vi "Asia Pump C Test.vi"() -> ()   [LabVIEW 2018, in "ASIA Pump.lvlib"]
uses:
  ASIA Pump.lvlib
  ASIA Pump/Pump Settings.ctl
panel:
  out "ASIA Pump Global 2":T1(array[cluster])
  out "ASIA Pump Global":T1(array[cluster])
  out "Set Speed Connection error":bool
  out "scan error out":errorcluster
  out "Initialized":bool
  out "No Pump Connected":bool=TRUE
  out "Enter Remote Completed":bool=TRUE
  in  "Enum":T2(ring)
  in  "stop 3":bool
  out "Set Overpressure Strategy":bool
  out "pumpCnt":u32
  in  "ASIA Pump C Settings in 3":T3={"ASIA Pump #"=0, "channel"=1, "Simulated"=FALSE}
  out "Pump On?":enum16{"Off", "On", "Not Initialized"}(ring)
  out "pressure":dbl
  out "Connection Error 2":bool
  out "Connection Error":bool
  out "Pump Status Time":dbl
  out "Set Speed Time":dbl
  in  "Pump %":sgl
  in  "stop":bool
  out "PumpStatusCode":T4(ring)=enum."Idle"
  out "pumpRate":dbl format="%.2f"
  out "syringeSize":sgl
  in  "Run":bool
  in  "ASIA Pump C Settings in":T3
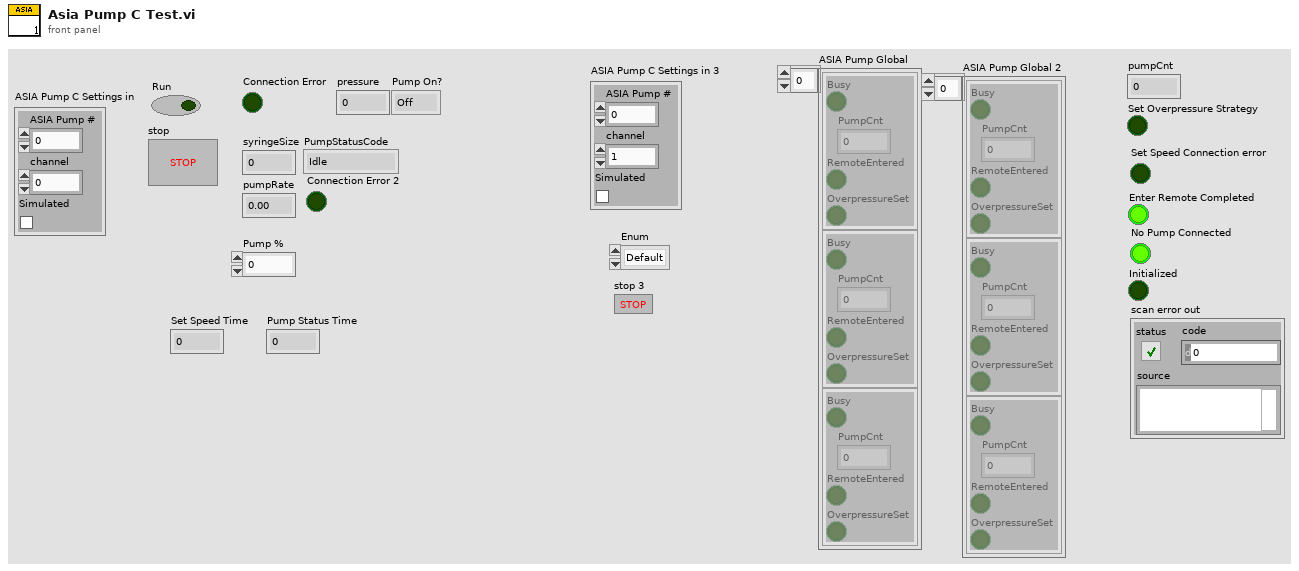
[diagram p1: front panel]
types:
  T1 = cluster{"Busy":bool, "PumpCnt":dbl, "RemoteEntered":bool, "OverpressureSet":bool}[]
  T2 = enum16{"Default", "EnterRemote", "Scan", "overpress", "initialize", "pump"}
  T3 = typedef "ASIA Pump.lvlib/Pump Settings.ctl" = cluster{"ASIA Pump #":i32, "channel":i32, "Simulated":bool}
  T4 = enum16{"Error", "Uninitialised", "Initialising", "Idle", "Filling", "Full", "Emptying", "Empty", "Pumping", "Default"}
  T5 = enum16{"Default", "EnterRemote", "Scan", "overpress"}
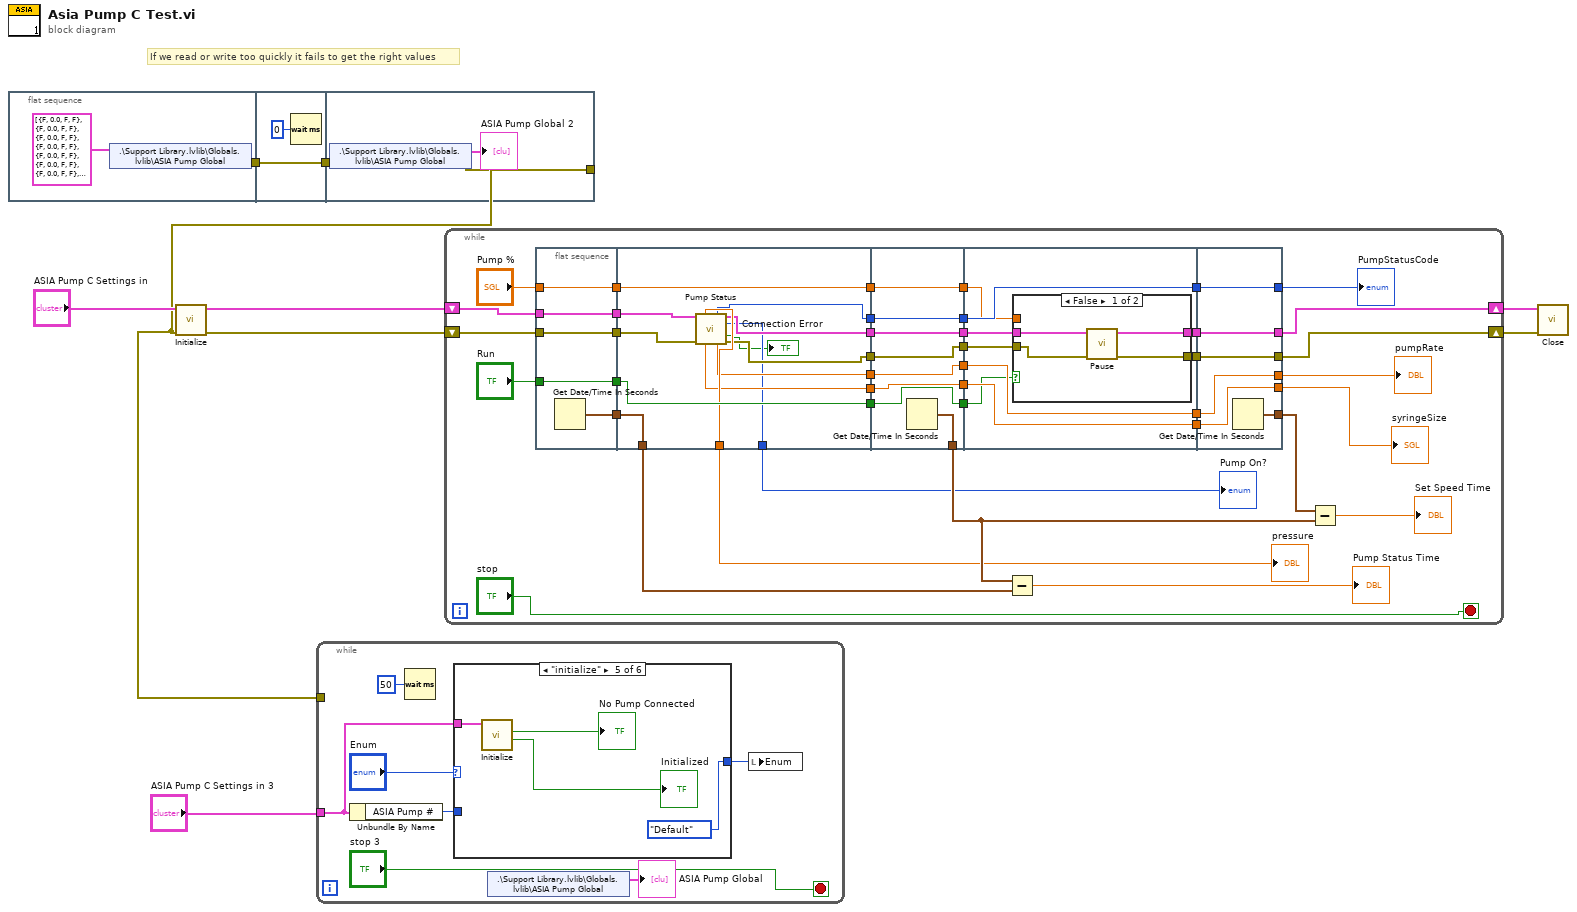
[diagram p0: block diagram]
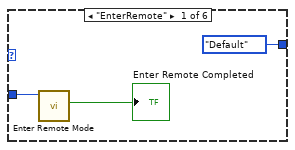
[diagram p2: hidden frame]
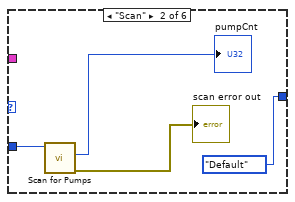
[diagram p3: hidden frame]
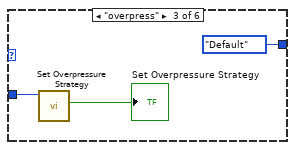
[diagram p4: hidden frame]
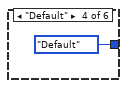
[diagram p5: hidden frame]
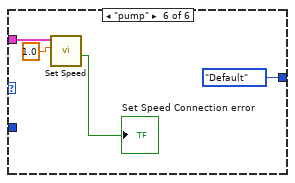
[diagram p6: hidden frame]
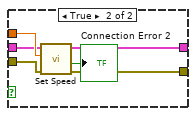
[diagram p7: hidden frame]
diagram:
  # "If we read or write too quickly it fails to get the right values"
  n1 = flat-sequence {
    tunnel: [w10] -> w3
    tunnel: w3 -> [w13]
    tunnel: [w13] -> w2
    tunnel: w2 -> [w15]
    tunnel: [w14] -> w1
    frame #0 {
      n2 = shared-variable ".\\Support Library.lvlib\\Globals.lvlib\\ASIA Pump Global"(T1 [{"Busy"=FALSE, "PumpCnt"=0.0, "RemoteEntered"=FALSE, "OverpressureSet"=FALSE}, {"Busy"=FALSE, "PumpCnt"=0.0, "RemoteEntered"=FALSE, "OverpressureSet"=FALSE}, {"Busy"=FALSE, "PumpCnt"=0.0, "RemoteEntered"=FALSE, "OverpressureSet"=FALSE}, {"Busy"=FALSE, "PumpCnt"=0.0, "RemoteEntered"=FALSE, "OverpressureSet"=FALSE}, {"Busy"=FALSE, "PumpCnt"=0.0, "RemoteEntered"=FALSE, "OverpressureSet"=FALSE}, {"Busy"=FALSE, "PumpCnt"=0.0, "RemoteEntered"=FALSE, "OverpressureSet"=FALSE}, {"Busy"=FALSE, "PumpCnt"=0.0, "RemoteEntered"=FALSE, "OverpressureSet"=FALSE}, {"Busy"=FALSE, "PumpCnt"=0.0, "RemoteEntered"=FALSE, "OverpressureSet"=FALSE}, {"Busy"=FALSE, "PumpCnt"=0.0, "RemoteEntered"=FALSE, "OverpressureSet"=FALSE}, {"Busy"=FALSE, "PumpCnt"=0.0, "RemoteEntered"=FALSE, "OverpressureSet"=FALSE}, {"Busy"=FALSE, "PumpCnt"=0.0, "RemoteEntered"=FALSE, "OverpressureSet"=FALSE}] ("ASIA Pump Global")) -> (error out=w10:errorcluster)  [unwired: 1 in]
    }
    frame #1 {
      n3 = Wait (ms)(milliseconds to wait=u32 0) -> ()  [unwired: 1 out]
    }
    frame #2 {
      n4 = shared-variable ".\\Support Library.lvlib\\Globals.lvlib\\ASIA Pump Global"(error in=w15) -> (→"ASIA Pump Global 2":T1, error out=w14:errorcluster)
    }
  }
  n5 = call "Initialize.vi"("error in (no error)"=w1, "ASIA Pump C Settings in"="ASIA Pump C Settings in") -> ("error out"=w5:errorcluster, "ASIA Pump C Settings out"=w8:T3)  [unwired: 6 in, 2 out]
  n6 = while {
    tunnel: "ASIA Pump C Settings in 3" -> [w19]
    tunnel: w1 -> [_]
    stop <- "stop 3" stop-if-true
    n7 = Unbundle By Name(w19) -> ("ASIA Pump #"=w23:i32)
    n8 = Wait (ms)(milliseconds to wait=u32 50) -> ()  [unwired: 1 out]
    n9 = case shown="\"initialize\"" "Enum" {
      tunnel: w23 -> [w25 w27 w31 _ _ _]
      tunnel: [T5."Default" T5."Default" T5."Default" T5."Default" T5."Default" T5."Default"] -> w20
      tunnel: w19 -> [_ _ _ _ w38 w41]
      frame "EnterRemote" {
        n10 = call "Enter Remote Mode.vi"("ASIA Pump #"=w25) -> ("Completed"=→"Enter Remote Completed":bool)  [unwired: 8 in, 2 out]
      }
      frame "Scan" {
        n11 = call "Scan for Pumps.vi"("ASIA Pump #"=w27) -> ("error out"=→"scan error out":errorcluster, "pumpCnt"=→"pumpCnt":u32)  [unwired: 8 in, 1 out]
      }
      frame "overpress" {
        n12 = call "Set Overpressure Strategy.vi"("ASIA Pump #"=w31) -> ("strategySet"=→"Set Overpressure Strategy":bool)  [unwired: 8 in, 2 out]
      }
      frame "Default" {
      }
      frame "initialize" {
        n13 = call "Initialize.vi"("ASIA Pump C Settings in"=w38) -> ("Initialized"=→"Initialized":bool, "No Pump Connected"=→"No Pump Connected":bool)  [unwired: 7 in, 2 out]
      }
      frame "pump" {
        n14 = call "Set Speed.vi"("Pump %"=sgl 1.0, "ASIA Pump C Settings in"=w41) -> ("Connection Error"=→"Set Speed Connection error":bool)  [unwired: 7 in, 2 out]
      }
    }
    n15 = shared-variable ".\\Support Library.lvlib\\Globals.lvlib\\ASIA Pump Global"() -> (→"ASIA Pump Global":T1)  [unwired: 1 in, 1 out]
    n16 = local write "Enum"(w20) -> ()
  }
  n17 = while {
    shift-right: [w82] -> w7
    shift-left: w8 -> [w83]
    shift-right: [w80] -> w6
    shift-left: w5 -> [w81]
    stop <- "stop" stop-if-true
    n18 = flat-sequence {
      tunnel: "Pump %" -> [w85]
      tunnel: "Run" -> [w86]
      tunnel: w81 -> [w87]
      tunnel: w83 -> [w88]
      tunnel: [w88] -> w72
      tunnel: [w87] -> w71
      tunnel: [w86] -> w70
      tunnel: [w85] -> w69
      tunnel: [w84] -> w68
      tunnel: [w94] -> w61
      tunnel: [w95] -> w59
      tunnel: [w91] -> w57
      tunnel: [w92] -> w55
      tunnel: w72 -> [w98]
      tunnel: w71 -> [w97]
      tunnel: w70 -> [w101]
      tunnel: w69 -> [w100]
      tunnel: w68 -> [w99]
      tunnel: [w101] -> w52
      tunnel: [w100] -> w50
      tunnel: [w99] -> w48
      tunnel: [w96] -> w45
      tunnel: [w90] -> w44
      tunnel: [w93] -> w43
      tunnel: w61 -> [w109]
      tunnel: [w109] -> w60
      tunnel: w59 -> [w108]
      tunnel: [w108] -> w58
      tunnel: w57 -> [w107]
      tunnel: [w107] -> w56
      tunnel: w55 -> [w106]
      tunnel: [w106] -> w54
      tunnel: [w105] -> w53
      tunnel: w52 -> [w104]
      tunnel: [w104] -> w51
      tunnel: w50 -> [w103]
      tunnel: [w103] -> w49
      tunnel: [w102] -> w46
      tunnel: w43 -> [w105]
      tunnel: w60 -> [w114]
      tunnel: [w111] -> w66
      tunnel: w58 -> [w113]
      tunnel: [w110] -> w65
      tunnel: w56 -> [w118]
      tunnel: [w118] -> w64
      tunnel: w54 -> [w117]
      tunnel: [w117] -> w63
      tunnel: w53 -> [w116]
      tunnel: [w116] -> w62
      tunnel: w51 -> [w115]
      tunnel: w49 -> [w112]
      tunnel: [w130] -> w76
      tunnel: [w131] -> w77
      tunnel: [w132] -> w78
      tunnel: [w133] -> w80
      tunnel: [w134] -> w82
      tunnel: w66 -> [w134]
      tunnel: w65 -> [w133]
      tunnel: w64 -> [w132]
      tunnel: w63 -> [w131]
      tunnel: w62 -> [w130]
      tunnel: [w129] -> w67
      frame #0 {
        n19 = Get Date/Time In Seconds() -> (seconds since 1Jan1904=w84:timestamp)
      }
      frame #1 {
        n20 = call "Pump Status.vi"("ASIA Pump C Settings in"=w98, "error in (no error)"=w97) -> ("pressure"=w96:dbl, "PumpStatusCode"=w93:T4, "ASIA Pump C Settings out"=w94:T3, "Pump On?"=w90:enum16{"Off", "On", "Not Initialized"}, "Connection Error"=→"Connection Error":bool, "syringeSize (ml)"=w91:sgl, "pumpRate"=w92:dbl, "error out"=w95:errorcluster)  [unwired: 5 in, 1 out]
      }
      frame #2 {
        n21 = Get Date/Time In Seconds() -> (seconds since 1Jan1904=w102:timestamp)
      }
      frame #3 {
        n22 = case shown="False" w115 {
          tunnel: w114 -> [w120 w125]
          tunnel: [w122 w128] -> w111
          tunnel: w113 -> [w119 w124]
          tunnel: [w121 w127] -> w110
          tunnel: w112 -> [_ w126]
          frame False {
            n23 = call "Pause.vi"("error in (no error)"=w119, "ASIA Pump C Settings in"=w120) -> ("error out"=w121:errorcluster, "ASIA Pump C Settings out"=w122:T3)  [unwired: 7 in, 1 out]
          }
          frame True {
            n24 = call "Set Speed.vi"("error in (no error)"=w124, "Pump %"=w126, "ASIA Pump C Settings in"=w125) -> ("error out"=w127:errorcluster, "Connection Error"=→"Connection Error 2":bool, "ASIA Pump C Settings out"=w128:T3)  [unwired: 6 in]
          }
        }
      }
      frame #4 {
        n25 = Get Date/Time In Seconds() -> (seconds since 1Jan1904=w129:timestamp)
      }
    }
    n26 = Subtract(x=w46, y=w48) -> (x-y=→"Pump Status Time":dbl)
    n27 = Subtract(x=w67, y=w46) -> (x-y=→"Set Speed Time":dbl)
    "syringeSize" <- w78
    "pumpRate" <- w77
    "PumpStatusCode" <- w76
    "pressure" <- w45
    "Pump On?" <- w44
  }
  n28 = call "Close.vi"("error in (no error)"=w6, "ASIA Pump C"=w7) -> ()  [unwired: 7 in, 3 out]
